vi "CRYStimulus File Path.vi"(11 "ViewTable":bool) -> (3 "FilePath":path)   [LabVIEW 2013]
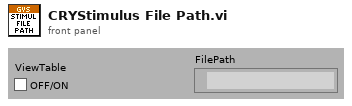
[diagram p1: front panel]
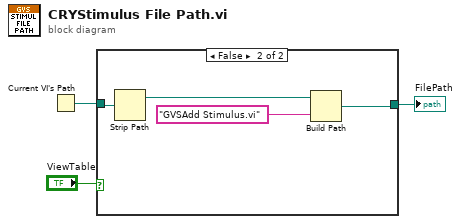
[diagram p0: block diagram]
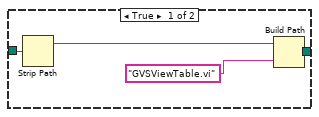
[diagram p2: hidden frame]
diagram:
  n1 = Current VI's Path() -> (path=w3:path)
  n2 = case shown="False" "ViewTable" {
    tunnel: w3 -> [w6 w10]
    tunnel: [w7 w11] -> w2
    frame True {
      n3 = Strip Path(path=w6) -> (stripped path=w5:path)  [unwired: 1 out]
      n4 = Build Path(base path=w5, name or relative path="GVSViewTable.vi" ("string")) -> (appended path=w7:path)
    }
    frame False, Default {
      n5 = Strip Path(path=w10) -> (stripped path=w9:path)  [unwired: 1 out]
      n6 = Build Path(base path=w9, name or relative path="GVSAdd Stimulus.vi" ("string")) -> (appended path=w11:path)
    }
  }
  "FilePath" <- w2
